vi "Configure Battery Emulator Capacity Limit.vi"(8 "error in (no error)":errorcluster, 10 "Value(0)":dbl, 11 "VISA resource name":refnum<visa-resource-name>) -> (0 "error out":errorcluster, 3 "VISA resource name out":refnum<visa-resource-name>)   [LabVIEW 2015, in "IT6000C.lvlib"]
doc: "This command sets the capacity of the battery simulation battery."
uses:
  <instrlib>/IT6000C/IT6000C.lvlib
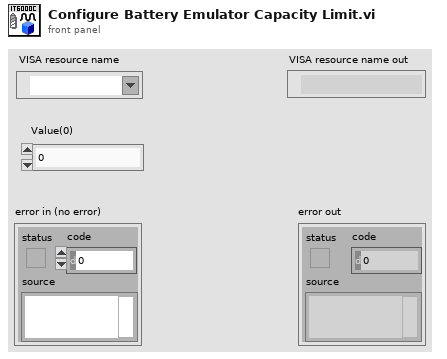
[diagram p1: front panel]
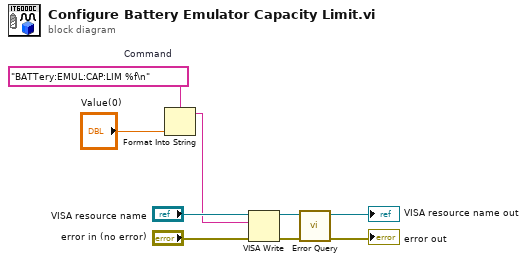
[diagram p0: block diagram]
diagram:
  w3 = "BATTery:EMUL:CAP:LIM %f\n"  # Command
  n1 = Format Into String(format string=w3, "Value(0)") -> (resulting string=w1:string)  [unwired: 2 in, 1 out]
  n2 = VISA Write(VISA resource name="VISA resource name", write buffer=w1, error in (no error)="error in (no error)") -> (VISA resource name out=w6:refnum<visa-resource-name>, error out=w7:errorcluster)  [unwired: 1 out]
  n3 = call <instrlib>:"Error Query.vi"("error in (no error)"=w7, "VISA resource name"=w6) -> ("error out"=→"error out":errorcluster, "VISA resource name out"=→"VISA resource name out":refnum<visa-resource-name>)  [unwired: 6 in, 2 out]
